vi "FTW-JSON-KeyExists.vi"(0 "JSON Object":refnum<class "FTW-JSON.lvclass">, 5 "Key":string, 11 "error in":errorcluster) -> (4 "JSON Object":refnum<class "FTW-JSON.lvclass">, 6 "Found?":bool, 15 "error out":errorcluster)   [LabVIEW 2013, in "FTW-JSON.lvclass"]
uses:
  FTW-JSON.lvclass
  FTW-JSON.lvclass/FTW-JSON.ctl
  lib/FTW-JSON-Type.ctl
panel:
  # "Inputs"
  # "Outputs"
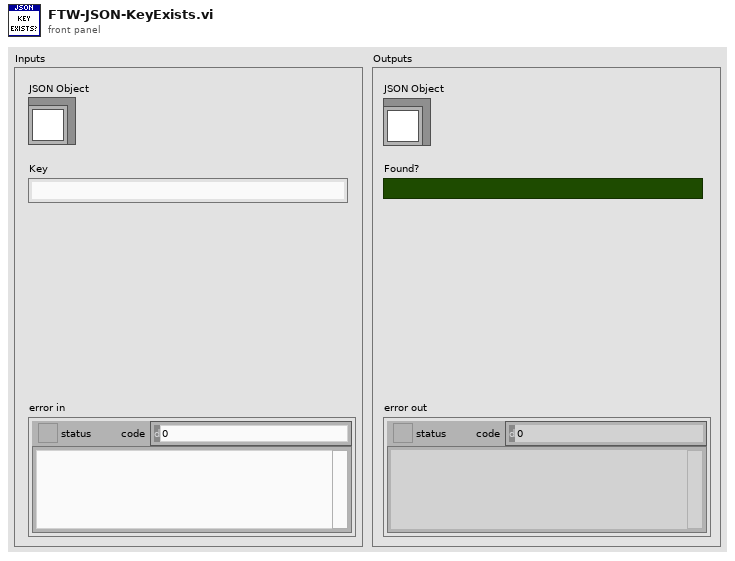
[diagram p1: front panel]
types:
  T1 = typedef "FTW-JSON-Type.ctl" = enum16{"Object", "Array", "String", "Integer", "Floating Point", "true", "false", "null", "undefined"}
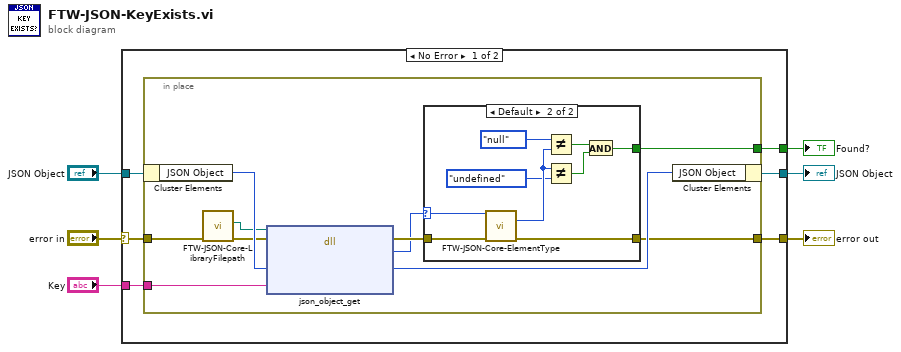
[diagram p0: block diagram]
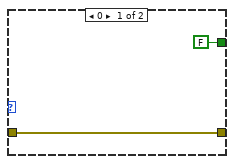
[diagram p2: hidden frame]
diagram:
  n1 = case shown="No Error" "error in" {
    selector: "error in" -> [w12 w35]
    tunnel: [w8 w35] -> w6
    tunnel: [w10 w34] -> w4
    tunnel: "JSON Object" -> [w11 w34]
    tunnel: "Key" -> [w9 _]
    tunnel: [w7 _] -> w1
    frame No Error {
      n2 = in-place {
        in-place-border: w12 -> [w22]
        in-place-border: w9 -> [w17]
        in-place-border: [w15] -> w8
        in-place-border: [w14] -> w7
        n3 = in-place-cluster #1(w11) -> ("JSON Object"=w21:i64)
        n4 = call "FTW-JSON-Core-LibraryFilepath.vi"("error in"=w22) -> ("error out"=w20:errorcluster, "JSON Library Filepath"=w19:path)  [unwired: 9 in]
        n5 = dll-call lib="?" fn="json_object_get"(path in=w19, error in=w20, "JSON Object Pointer"=w21, "Element Key"=w17) -> (error out=w16:errorcluster, "JSON Element Pointer"=w13:i64, "JSON Object Pointer"=w18:i64)  [unwired: 2 in, 1 out]
        n6 = case shown="Default" w13 {
          selector: w13 -> [_ w25]
          tunnel: w16 -> [w24 w33]
          tunnel: [w24 w32] -> w15
          tunnel: [FALSE w30] -> w14
          frame 0 {
          }
          frame Default {
            n7 = call "FTW-JSON-Core-ElementType.vi"("JSON Element"=w25, "error in"=w33) -> ("JSON Type"=w29:T1, "error out"=w32:errorcluster)  [unwired: 11 in, 1 out]
            n8 = Not Equal?(x=FTW-JSON-Type."null", y=w29) -> (x != y?=w28:bool)
            n9 = Not Equal?(x=w29, y=FTW-JSON-Type."undefined") -> (x != y?=w27:bool)
            n10 = And(x=w28, y=w27) -> (x .and. y?=w30:bool)
          }
        }
        n11 = in-place-cluster #1("JSON Object"=w18) -> (w10:refnum<class "FTW-JSON.lvclass">)
      }
    }
    frame Error {
    }
  }
  "error out" <- w6
  "JSON Object" <- w4
  "Found?" <- w1
